vi "Occurence-Trigger.vi"(2 "Done":refnum<k4>, 9 "error in (no error)":errorcluster) -> (6 "error out":errorcluster)   [LabVIEW 2009]
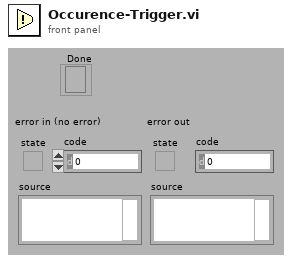
[diagram p1: front panel]
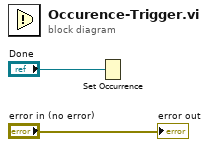
[diagram p0: block diagram]
diagram:
  n1 = Set Occurrence("Done") -> ()
  "error out" <- "error in (no error)"
